vi "Launcher.vi"() -> ()   [LabVIEW 2021]
uses:
  Task Base/Task Base.lvclass
panel:
  out "Task":string[](array[string])
  out "Item Names":string[][](array[string])
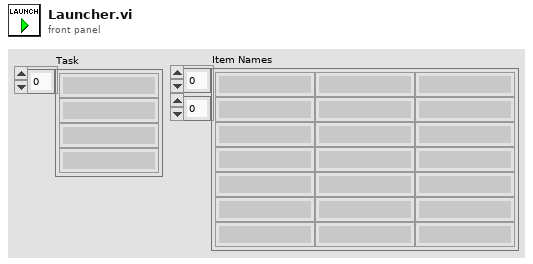
[diagram p1: front panel]
types:
  T1 = map{string, refnum<class "Build_Javier_Lopez_lib_Configuration_Filejson class.lvclass">}
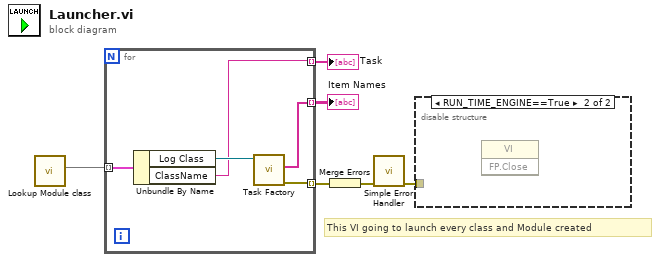
[diagram p0: block diagram]
diagram:
  # "This VI going to launch every class and Module created"
  n1 = call "Lookup Module class.vi"() -> ("Enum"=w6:T1)  [unwired: 10 in, 1 out]
  n2 = for {
    tunnel: w6 -> [w11] mode=indexing
    tunnel: [w9] -> w4 mode=indexing
    tunnel: [w7] -> w2 mode=indexing
    tunnel: [w8] -> w1 mode=indexing
    n3 = Unbundle By Name(w11) -> ("Log Class"=w10:refnum<class "Build_Javier_Lopez_lib_Configuration_Filejson class.lvclass">, "ClassName"=w8:string)
    n4 = call "Task Factory.vi"("Task Ref"=w10) -> ("error out"=w9:errorcluster, "Item Names"=w7:string[])  [unwired: 9 in]
  }
  "Item Names" <- w2
  "Task" <- w1
  n5 = Merge Errors(w4) -> (w5:errorcluster)
  n6 = call <vilib>:"Simple Error Handler.vi"("error in (no error)"=w5) -> ("error out"=w3:errorcluster)  [unwired: 4 in, 4 out]
  n7 = disable-structure shown="RUN_TIME_ENGINE==True" {
    disable-tunnel: w3 -> [_ _]
    frame condition #0 (active) {
    }
    frame condition #1 {
      n8 = invoke class="VI" method="FP.Close"() -> ()  [unwired: 3 in, 3 out]
    }
  }
